vi "Global Variables.vi"() -> ()   [LabVIEW 2014]
panel:
  in  "Eject Encoder":string
  in  "Lift encoder":string
  in  "Eject?":string
  in  "Lift Top":string
  in  "Lift Home":string
  in  "Tote Sensor":string
  in  "Gyro":string
  in  "Door Right":string
  in  "Door Left":string
  in  "Roller Move Right":string
  in  "Roller Move Left":string
  in  "Eject":string
  in  "Roller Right":string
  in  "Roller Left":string
  in  "Chain Lift":string
  in  "Rotational Motor BR":string
  in  "Rotational Motor FL":string
  in  "Rotational Motor BL":string
  in  "Rotational Motor FR":string
  in  "V Encoder BL":string
  in  "V Encoder BR":string
  in  "V Encoder FL":string
  in  "V Encoder FR":string
  in  "A Encoder BL":string
  in  "A Encoder BR":string
  in  "A Encoder FL":string
  in  "A Encoder FR":string
  in  "Joystick R 1":string
  in  "Joystick L 1":string
  in  "Drive BL":string
  in  "Drive BR":string
  in  "Drive FL":string
  in  "Drive FR":string
  in  "Pivots Enabled?":bool
  in  "Calibration BR":dbl
  in  "Calibration BL":dbl
  in  "Calibration FR":dbl
  in  "Calibration FL":dbl
  in  "Rot Motor BR":dbl
  in  "Rot Motor BL":dbl
  in  "Rot Motor FR":dbl
  in  "Rot Motor FL":dbl
  in  "Drive Motor BR":dbl
  in  "Drive Motor BL":dbl
  in  "Drive Motor FR":dbl
  in  "Drive Motor FL":dbl
  # "Booleans"
  # "Values"
  # "Strings"
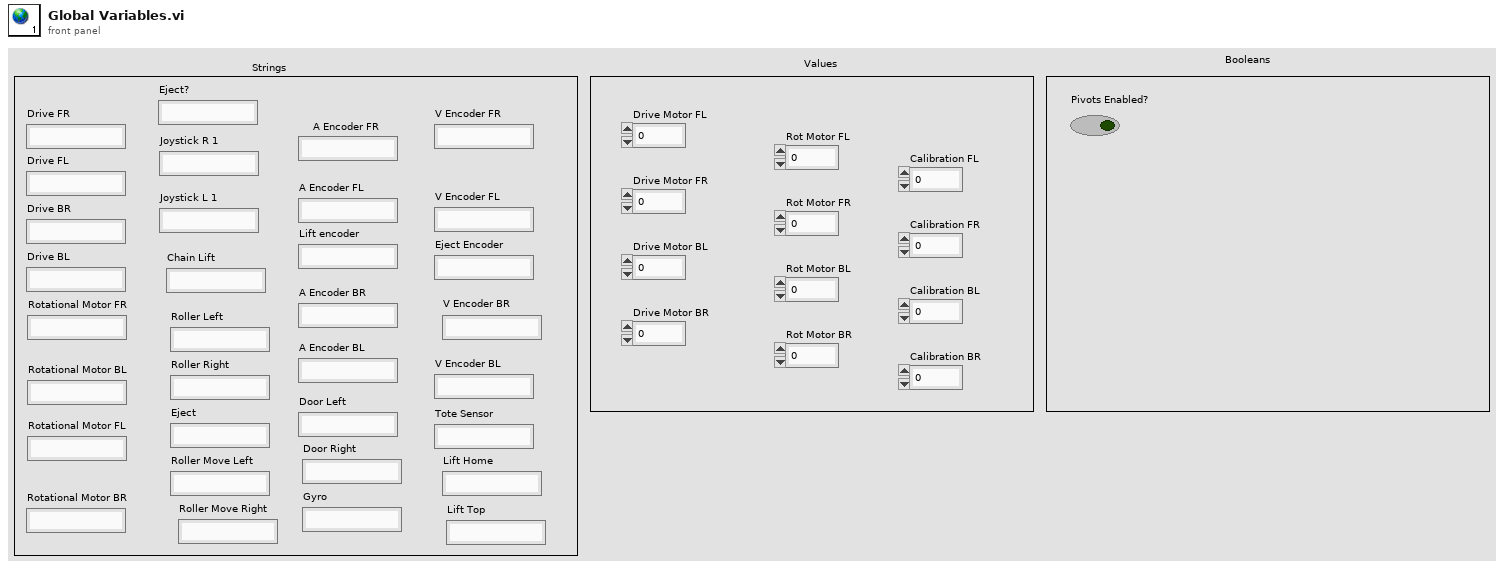
[diagram p1: front panel]
diagram:
